vi "InitFFT_result.vi"(10 "N average":i32=3 min=1, 11 "sequence IN":T2) -> (1 "initialized frame array":dbl[][](array[numeric]), 2 "initialized FFT array":cdb[][](array[numeric]), 3 "fft cluster":T1, 6 "Stot":i32)   [LabVIEW 2018]
uses:
  General Libraries/myFFT.lvlib
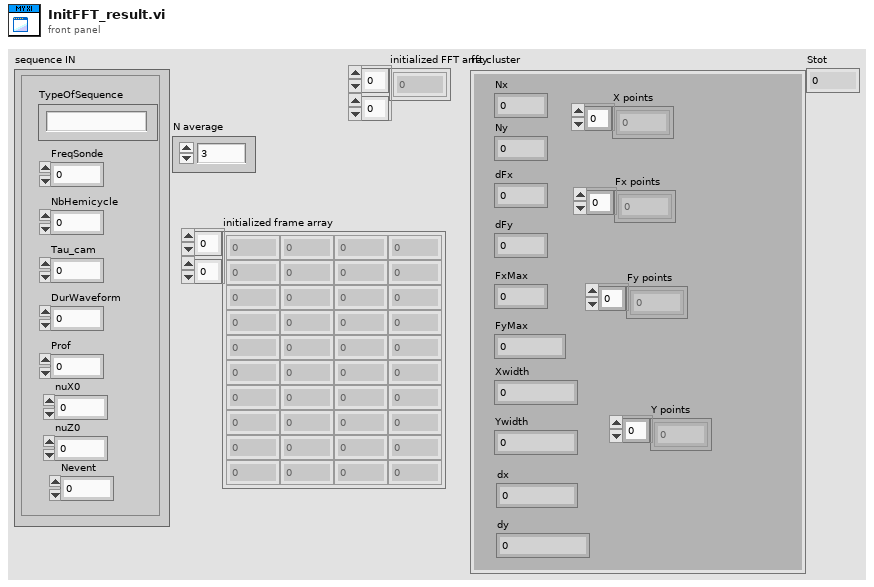
[diagram p1: front panel]
types:
  T1 = cluster{"dFx":dbl, "dFy":dbl, "Nx":i32, "Ny":i32, "FxMax":dbl, "FyMax":dbl, "Xwidth":dbl, "Ywidth":dbl, "dx":dbl, "dy":dbl, "Fx points":dbl[], "X points":dbl[], "Y points":dbl[], "Fy points":dbl[]}
  T2 = cluster{"TypeOfSequence":string, "FreqSonde":dbl, "NbHemicycle":dbl, "Tau_cam":dbl, "DurWaveform":dbl, "Prof":dbl, "Nevent":i32, "nuX0":dbl, "nuZ0":dbl}
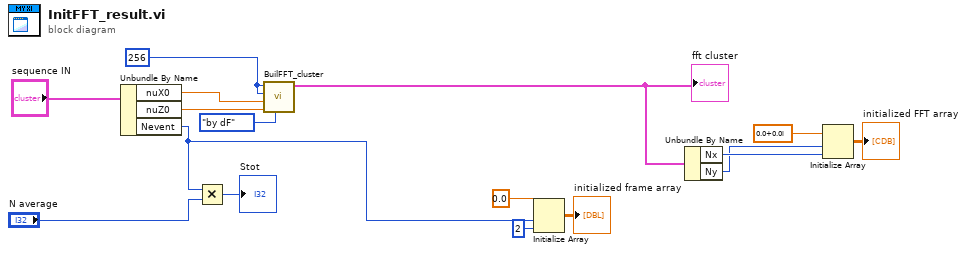
[diagram p0: block diagram]
diagram:
  w15 = 256 ("dimension size")
  n1 = Unbundle By Name("sequence IN") -> ("nuX0"=w14:dbl, "nuZ0"=w13:dbl, "Nevent"=w3:i32)
  n2 = Multiply(x=w3, y="N average") -> (x*y=→"Stot":i32)
  n3 = call "BuilFFT_cluster.vi"("Enum"=enum16{"by dF", "by dX"}."by dF", "input Y"=w13, "input X"=w14, "Ny"=w15, "Nx"=w15) -> ("fft cluster"=w10:T1)  [unwired: 6 in]
  "fft cluster" <- w10
  n4 = Initialize Array(0.0, w3, 2 ("dimension size")) -> (→"initialized frame array":dbl[][])
  n5 = Unbundle By Name(w10) -> ("Nx"=w9:i32, "Ny"=w8:i32)
  n6 = Initialize Array(cdb 0.0+0.0i ("element"), w8, w9) -> (→"initialized FFT array":cdb[][])
